vi "ImageStiching.vi"() -> ()   [LabVIEW 2019]
uses:
  <vilib>/userDefined/High Color/IMAQdx.ctl
  <vilib>/vision/NI_Vision_Development_Module.lvlib
panel:
  in  "error in (no error)":errorcluster
  in  "BackToInitail":string="G91\nG1 X-1.6703 Y-1.3974 F100"
  in  "ImageX2Y2":string="G91\nG1 X1.6703 Y0 F100"
  in  "ImageX1Y1":string="G91\nG1 X-1.6703 Y1.3974 F100"
  in  "ImageX2Y1":string="G91\nG1 X1.6703 Y0 F100"
  out "StichedImage2x2":T1(plugin-control)
  out "error out":errorcluster
  out "Image":T1[](array[plugin-control])
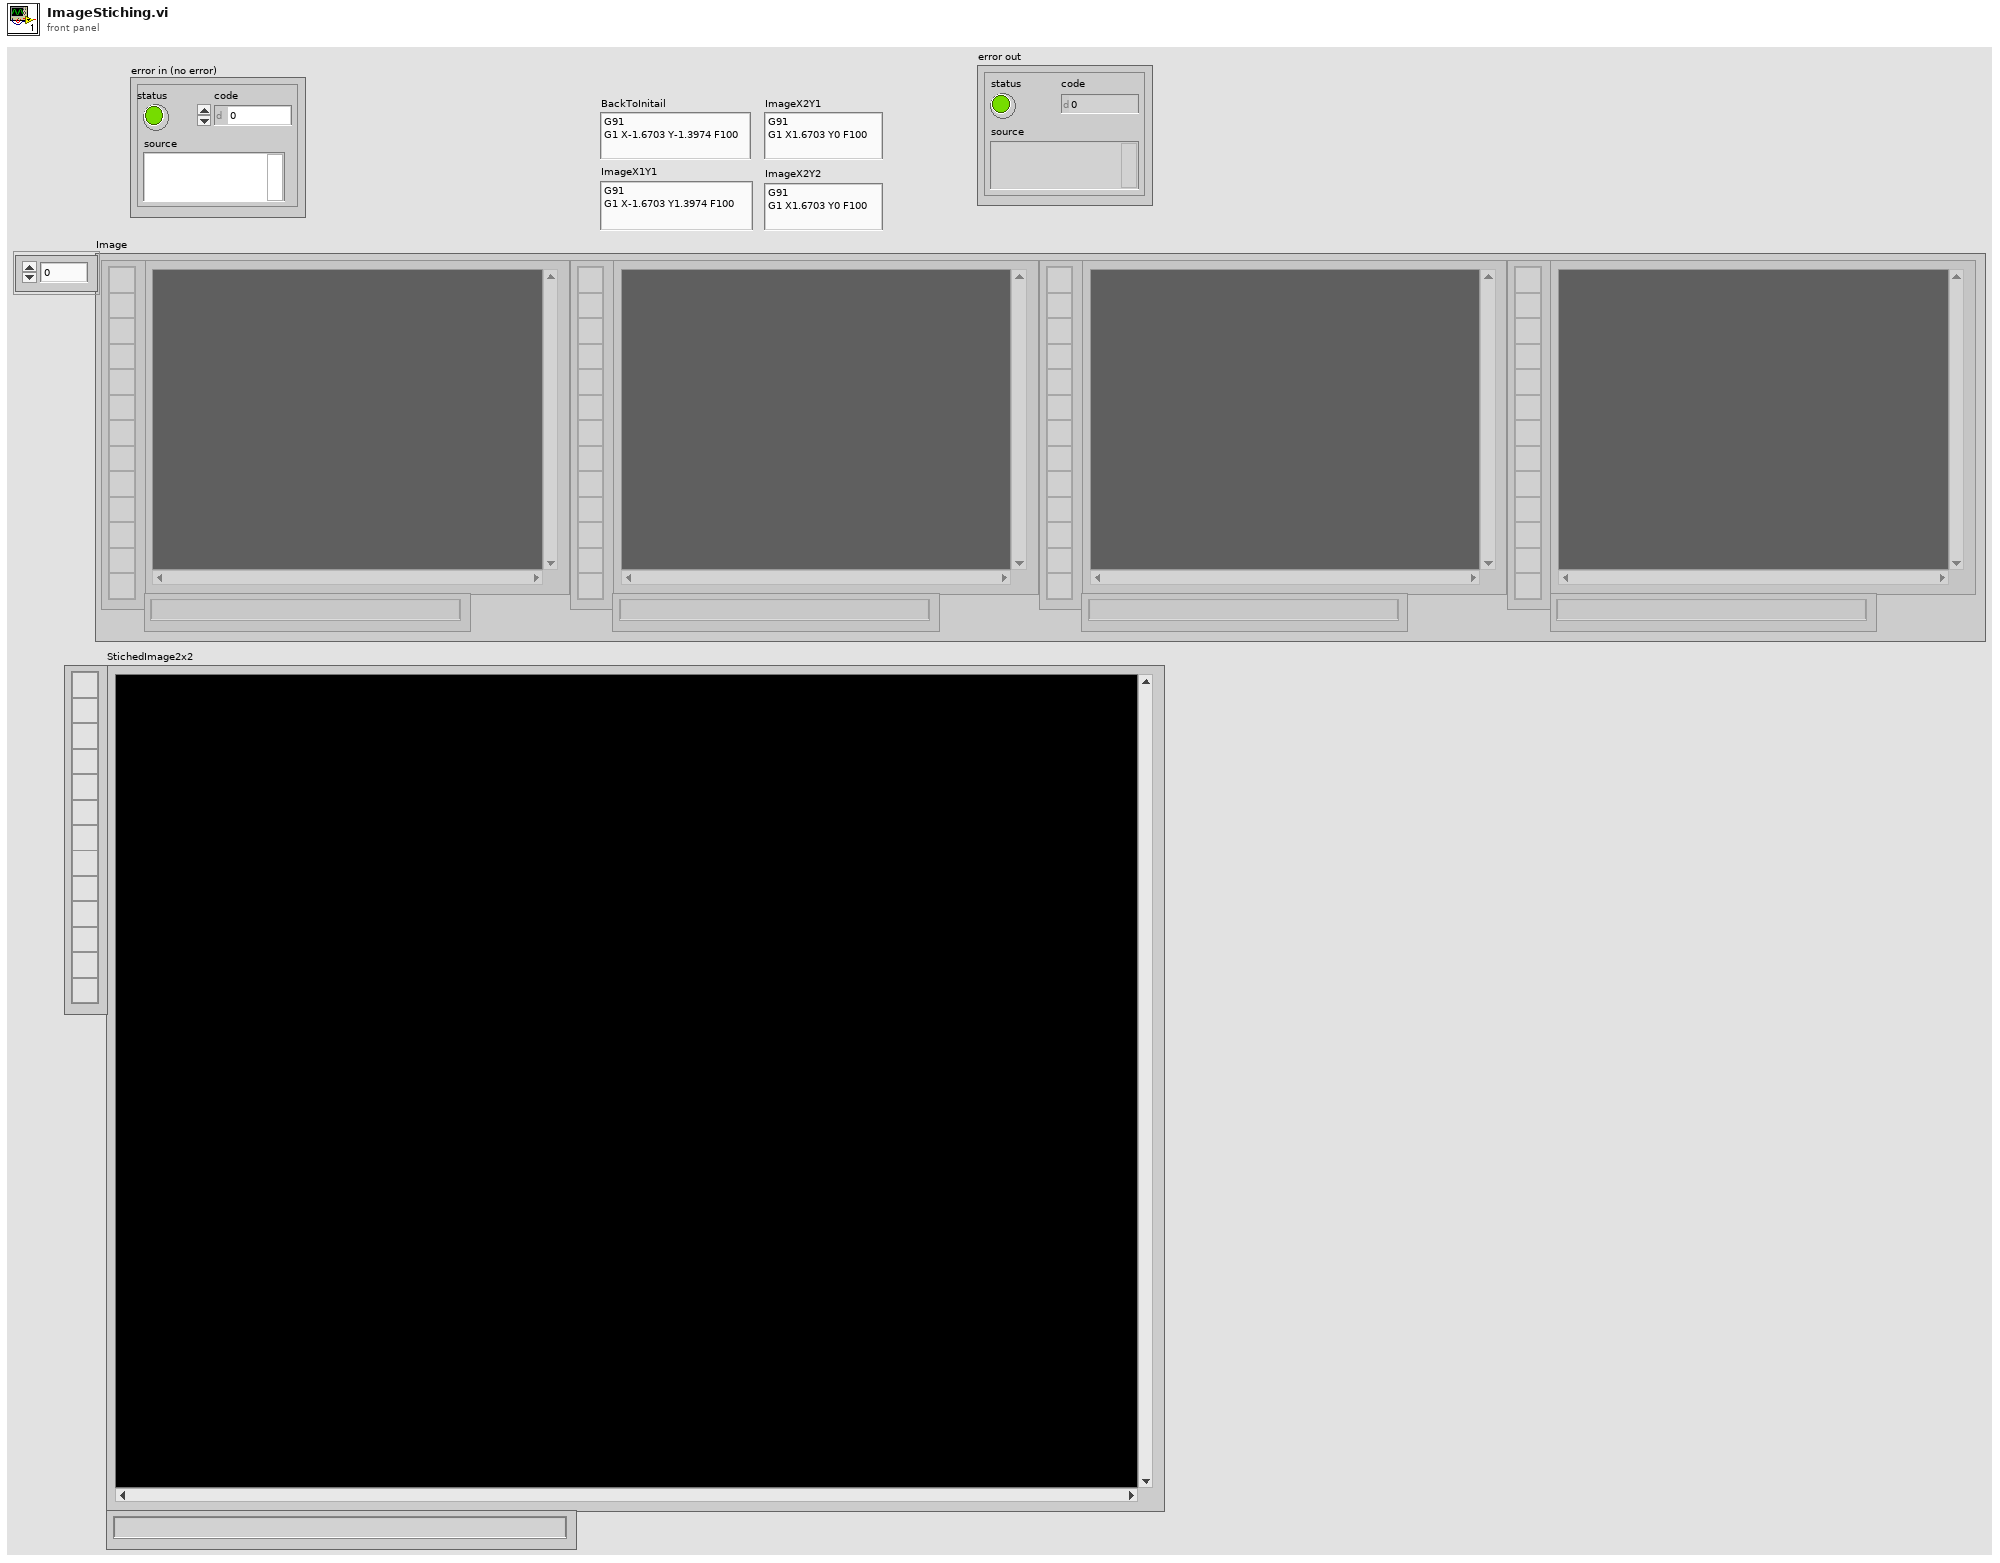
[diagram p1: front panel]
types:
  T1 = typedef "IMAQ Image.ctl" = refnum<image>
  T2 = typedef "IMAQdx.ctl" = refnum<k21>
  T3 = typedef "Image Type" = u32
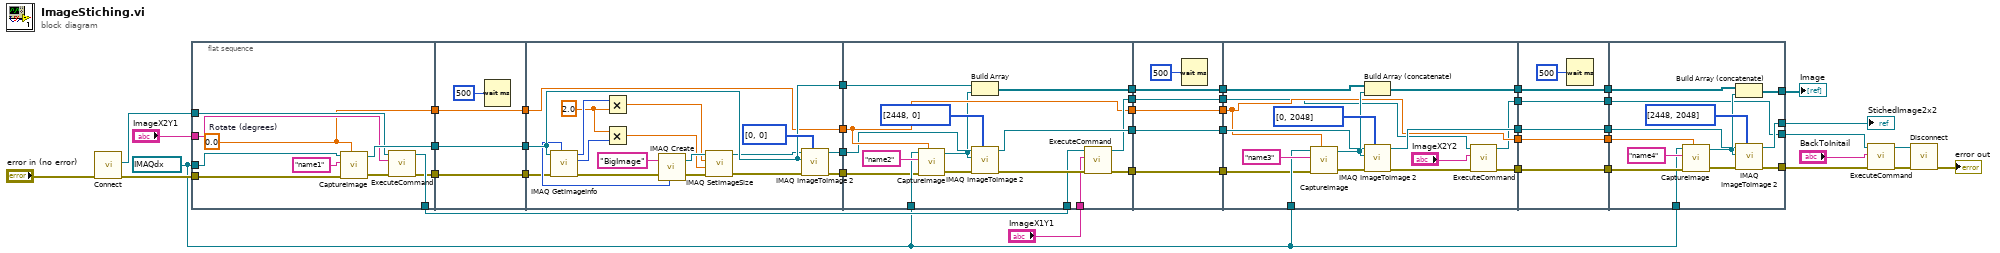
[diagram p0: block diagram]
diagram:
  w6 = T2 "cam1" ("Camera")
  n1 = call "Connect.vi"("error in (no error)"="error in (no error)") -> ("error out"=w42:errorcluster, "controller"=w39:refnum<k24>)  [unwired: 9 in]
  n2 = flat-sequence {
    tunnel: w6 -> [w54]
    tunnel: [w53] -> w41
    tunnel: w42 -> [w52]
    tunnel: w39 -> [w50]
    tunnel: "ImageX2Y1" -> [w49]
    tunnel: [w48] -> w32
    tunnel: [w47] -> w37
    tunnel: [w46] -> w33
    tunnel: w41 -> [w59]
    tunnel: [w59] -> w40
    tunnel: [w57] -> w38
    tunnel: w37 -> [w57]
    tunnel: [w56] -> w34
    tunnel: w33 -> [w56]
    tunnel: w40 -> [w73]
    tunnel: [w75] -> w45
    tunnel: [w73] -> w44
    tunnel: [w74] -> w43
    tunnel: w38 -> [w65]
    tunnel: [w64] -> w35
    tunnel: w34 -> [w64]
    tunnel: "ImageX1Y1" -> [w90]
    tunnel: w32 -> [w89]
    tunnel: [w93] -> w30
    tunnel: [w92] -> w28
    tunnel: [w88] -> w26
    tunnel: [w87] -> w24
    tunnel: [w86] -> w21
    tunnel: w35 -> [w86]
    tunnel: w43 -> [w79]
    tunnel: w44 -> [w83]
    tunnel: w45 -> [w82]
    tunnel: w6 -> [w84]
    tunnel: w30 -> [w99]
    tunnel: [w99] -> w29
    tunnel: w28 -> [w98]
    tunnel: [w98] -> w27
    tunnel: w26 -> [w97]
    tunnel: [w97] -> w25
    tunnel: w24 -> [w96]
    tunnel: [w96] -> w23
    tunnel: [w94] -> w22
    tunnel: w21 -> [w94]
    tunnel: w29 -> [w110]
    tunnel: w27 -> [w111]
    tunnel: w25 -> [w108]
    tunnel: w23 -> [w104]
    tunnel: w6 -> [w109]
    tunnel: w22 -> [w105]
    tunnel: [w107] -> w14
    tunnel: [w101] -> w13
    tunnel: [w103] -> w12
    tunnel: [w106] -> w11
    tunnel: [w105] -> w7
    tunnel: w14 -> [w116]
    tunnel: w13 -> [w121]
    tunnel: w12 -> [w117]
    tunnel: w11 -> [w120]
    tunnel: [w121] -> w10
    tunnel: [w120] -> w9
    tunnel: [w118] -> w8
    tunnel: w7 -> [w118]
    tunnel: [w117] -> w3
    tunnel: [w116] -> w2
    tunnel: [w125] -> w5
    tunnel: [w123] -> w18
    tunnel: [w126] -> w16
    tunnel: w10 -> [w129]
    tunnel: w9 -> [w130]
    tunnel: w8 -> [w128]
    tunnel: w6 -> [w127]
    tunnel: [w124] -> w4
    tunnel: w3 -> [w123]
    tunnel: w2 -> [w122]
    frame #0 {
      w46 = sgl 0.0  # Rotate (degrees)
      n3 = call "CaptureImage.vi"("Camera"=w54, "Rotate (degrees)"=w46, "ImageName"="name1", "error in (no error)"=w52) -> ("Image"=w53:T1, "error out"=w51:errorcluster)  [unwired: 3 in]
      n4 = call "ExecuteCommand.vi"("error in (no error)"=w51, "Command Code"=w49, "controller in"=w50) -> ("error out"=w47:errorcluster, "controller out"=w48:refnum<k24>)  [unwired: 6 in, 1 out]
    }
    frame #1 {
      n5 = Wait (ms)(milliseconds to wait=u32 500) -> ()  [unwired: 1 out]
    }
    frame #2 {
      w60 = 2.0 ("y")
      n6 = call "IMAQ GetImageInfo"("error in (no error)"=w65, "Image"=w73) -> ("error out"=w63:errorcluster, "Y Resolution"=w61:i32, "X Resolution"=w67:i32, "Image Type"=w72:T3)  [unwired: 2 in, 4 out]
      n7 = Multiply(x=w67, y=w60) -> (x*y=w66:dbl)
      n8 = Multiply(x=w60, y=w61) -> (x*y=w62:dbl)
      n9 = call "IMAQ Create"("Image Name"="BigImage", "Image Type"=w72, "error in (no error)"=w63) -> ("New Image"=w69:T1, "error out"=w71:errorcluster)  [unwired: 2 in]
      n10 = call "IMAQ SetImageSize"("error in (no error)"=w71, "Y Resolution"=w62, "X Resolution"=w66, "Image"=w69) -> ("error out"=w70:errorcluster, "Image Out"=w68:T1)  [unwired: 1 out]
      n11 = call "IMAQ ImageToImage 2"("Offset Left/Top"=i32[] [0, 0], "error in (no error)"=w70, "Image Src (Small)"=w73, "Image Src (Large)"=w68) -> ("error out"=w75:errorcluster, "Image Dst Out"=w74:T1)  [unwired: 2 in, 4 out]
    }
    frame #3 {
      n12 = call "CaptureImage.vi"("Camera"=w84, "Rotate (degrees)"=w86, "ImageName"="name2", "error in (no error)"=w82) -> ("Image"=w78:T1, "error out"=w80:errorcluster)  [unwired: 3 in]
      n13 = Build Array(w83, w78) -> (w93:T1[])
      n14 = call "IMAQ ImageToImage 2"("Offset Left/Top"=i32[] [2448, 0], "error in (no error)"=w80, "Image Src (Small)"=w78, "Image Src (Large)"=w79) -> ("error out"=w91:errorcluster, "Image Dst Out"=w92:T1)  [unwired: 2 in, 4 out]
      n15 = call "ExecuteCommand.vi"("error in (no error)"=w91, "Command Code"=w90, "controller in"=w89) -> ("error out"=w88:errorcluster, "controller out"=w87:refnum<k24>)  [unwired: 6 in, 1 out]
    }
    frame #4 {
      n16 = Wait (ms)(milliseconds to wait=u32 500) -> ()  [unwired: 1 out]
    }
    frame #5 {
      n17 = call "CaptureImage.vi"("Camera"=w109, "Rotate (degrees)"=w105, "ImageName"="name3", "error in (no error)"=w108) -> ("Image"=w112:T1, "error out"=w113:errorcluster)  [unwired: 3 in]
      n18 = Build Array (concatenate)(w110, w112) -> (w106:T1[])
      n19 = call "IMAQ ImageToImage 2"("Offset Left/Top"=i32[] [0, 2048], "error in (no error)"=w113, "Image Src (Small)"=w112, "Image Src (Large)"=w111) -> ("error out"=w102:errorcluster, "Image Dst Out"=w107:T1)  [unwired: 2 in, 4 out]
      n20 = call "ExecuteCommand.vi"("error in (no error)"=w102, "Command Code"="ImageX2Y2", "controller in"=w104) -> ("error out"=w101:errorcluster, "controller out"=w103:refnum<k24>)  [unwired: 6 in, 1 out]
    }
    frame #6 {
      n21 = Wait (ms)(milliseconds to wait=u32 500) -> ()  [unwired: 1 out]
    }
    frame #7 {
      n22 = call "CaptureImage.vi"("Camera"=w127, "Rotate (degrees)"=w128, "ImageName"="name4", "error in (no error)"=w129) -> ("Image"=w131:T1, "error out"=w132:errorcluster)  [unwired: 3 in]
      n23 = Build Array (concatenate)(w130, w131) -> (w124:T1[])
      n24 = call "IMAQ ImageToImage 2"("Offset Left/Top"=i32[] [2448, 2048], "error in (no error)"=w132, "Image Src (Small)"=w131, "Image Src (Large)"=w122) -> ("error out"=w126:errorcluster, "Image Dst Out"=w125:T1)  [unwired: 2 in, 4 out]
    }
  }
  n25 = call "ExecuteCommand.vi"("error in (no error)"=w16, "Command Code"="BackToInitail", "controller in"=w18) -> ("error out"=w15:errorcluster, "controller out"=w17:refnum<k24>)  [unwired: 6 in, 1 out]
  n26 = call "Disconnect.vi"("error in (no error)"=w15, "controller"=w17) -> ("error out"=→"error out":errorcluster)  [unwired: 9 in]
  "Image" <- w4
  "StichedImage2x2" <- w5
